vi "Set Run Control.vi"(8 "error in (no error)":errorcluster, 10 "Run Control":T1, 11 "PXIe5105 in":refnum<class "PXIe5105.lvclass">) -> (0 "error out":errorcluster, 3 "PXIe5105 out":refnum<class "PXIe5105.lvclass">)   [LabVIEW 2018, in "PXIe5105.lvlib" / "PXIe5105.lvclass"]
doc: "This Override method is used to set the Oscope instrument running mode. The 'Run Control' control has 3 modes of operation: 0-Run (or continuous), 1 - Single, 2 - Stop."
uses:
  PXIe5105.lvclass
  PPLs/Oscilloscope/Parent/Oscilloscope.lvlibp/Custom Controls/Run Control.ctl
  PXIe5105.lvclass/PXIe5105.ctl
  <instrlib>/niScope/Configure/Trigger/niScope Configure Trigger Software.vi
  PPLs/Oscilloscope/Parent/Oscilloscope.lvlibp
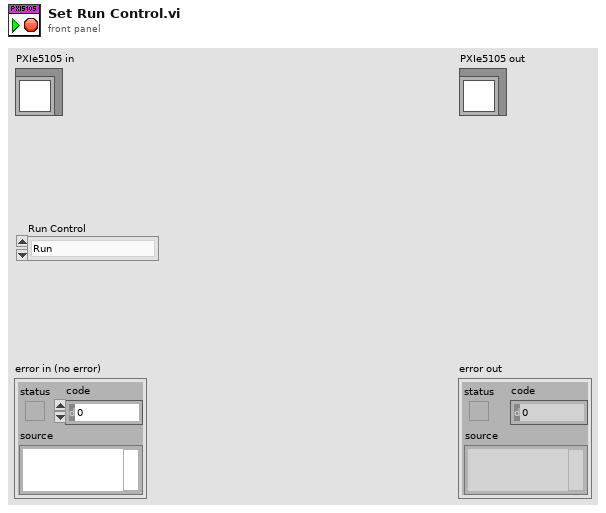
[diagram p1: front panel]
types:
  T1 = typedef "Oscilloscope.lvlibp/Run Control.ctl" = enum16{"Run", "Single", "Stop"}
  T2 = typedef "Oscilloscope.lvlibp/Analog Channels.ctl" = enum16{"1", "2", "3", "4", "5", "6", "7", "8", "9", "10", "11", "12", "13", "14", "15", "16"}
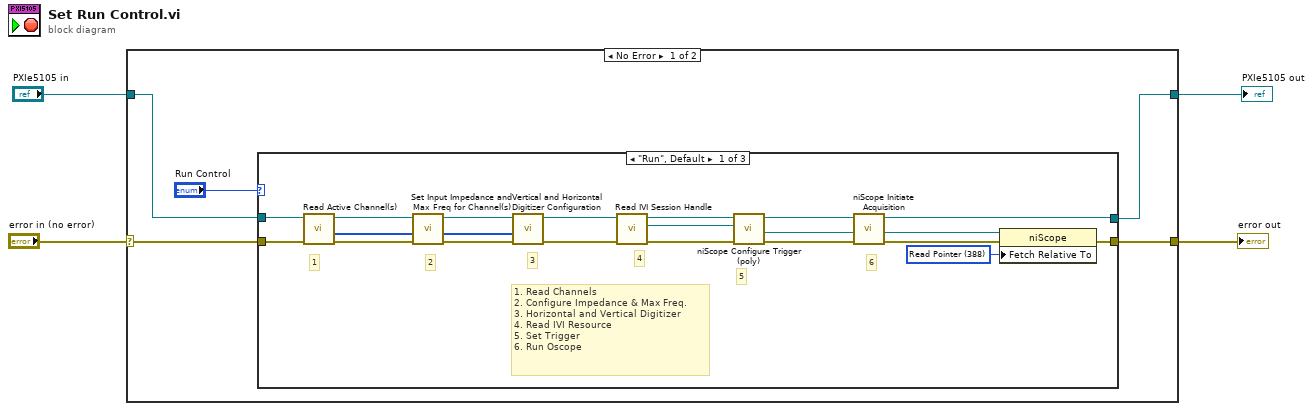
[diagram p0: block diagram]
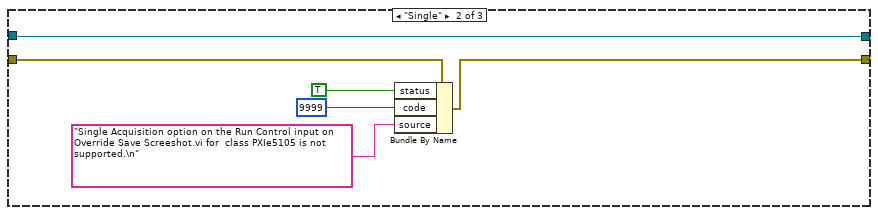
[diagram p2: hidden frame]
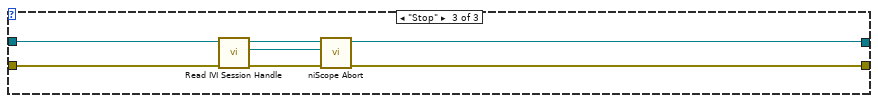
[diagram p3: hidden frame]
diagram:
  n1 = case shown="No Error" "error in (no error)" {
    selector: "error in (no error)" -> [w7 w41]
    tunnel: [w8 w41] -> w3
    tunnel: [w5 w40] -> w2
    tunnel: "PXIe5105 in" -> [w6 w40]
    frame No Error {
      n2 = case shown="\"Run\", Default" "Run Control" {
        tunnel: w7 -> [w26 w30 w36]
        tunnel: [w12 w29 w39] -> w8
        tunnel: w6 -> [w27 w28 w38]
        tunnel: [w19 w28 w34] -> w5
        frame "Run", Default {
          w15 = 388 items=["Start"=482, "Trigger"=483, "Pretrigger"=477, "Now"=481, "Read Pointer"=388] ("Fetch:Fetch Relative To")
          # "6"
          # "1. Read Channels\n2. Configure Impedance & Max Freq.\n3. Horizontal and Vertical Digitizer\n4. Read IVI Resource\n5. Set Trigger\n6. Run Oscope"
          # "5"
          # "4"
          # "3"
          # "2"
          # "1"
          n3 = call "Read Active Channel(s).vi"("error in (no error)"=w26, "PXIe5105 in"=w27) -> ("error out"=w25:errorcluster, "Active Channel(s)"=w18:T2[], "PXIe5105 out"=w23:refnum<class "PXIe5105.lvclass">)  [unwired: 7 in]
          n4 = call "Set Input Impedance and Max Freq for Channel(s).vi"("Channel(s)"=w18, "error in (no error)"=w25, "PXIe5105 in"=w23) -> ("error out"=w24:errorcluster, "PXIe5105 out"=w22:refnum<class "PXIe5105.lvclass">)  [unwired: 7 in]
          n5 = call "Vertical and Horizontal Digitizer Configuration.vi"("Channel(s)"=w18, "error in (no error)"=w24, "PXIe5105 in"=w22) -> ("error out"=w20:errorcluster, "PXIe5105 out"=w21:refnum<class "PXIe5105.lvclass">)  [unwired: 7 in]
          n6 = call "Read IVI Session Handle.vi"("error in (no error)"=w20, "PXIe5105 in"=w21) -> ("error out"=w16:errorcluster, "IVI Session Handle"=w17:refnum<k15>, "PXIe5105 out"=w19:refnum<class "PXIe5105.lvclass">)  [unwired: 7 in]
          n7 = call-poly <instrlib>:"niScope Configure Trigger (poly).vi"("instrument handle"=w17, "error in"=w16) -> ("instrument handle out"=w11:refnum<k15>, "error out"=w14:errorcluster)  [unwired: 12 in]
          n8 = call <instrlib>:"niScope Initiate Acquisition.vi"("instrument handle"=w11, "error in"=w14) -> ("instrument handle out"=w10:refnum<k15>, "error out"=w13:errorcluster)  [unwired: 12 in]
          n9 = property class="niScope"(reference=w10, error in=w13, "Fetch Relative To"=w15) -> (error out=w12:errorcluster)  [unwired: 1 out]
        }
        frame "Single" {
          n10 = Bundle By Name(cluster=w30, "status"=TRUE, "code"=9999, "source"="Single Acquisition option on the Run Control input on Override Save Screeshot.vi for  class PXIe5105 is not supported.\n") -> (w29:errorcluster)
        }
        frame "Stop" {
          n11 = call "Read IVI Session Handle.vi"("error in (no error)"=w36, "PXIe5105 in"=w38) -> ("error out"=w35:errorcluster, "IVI Session Handle"=w37:refnum<k15>, "PXIe5105 out"=w34:refnum<class "PXIe5105.lvclass">)  [unwired: 7 in]
          n12 = call <instrlib>:"niScope Abort.vi"("instrument handle"=w37, "error in"=w35) -> ("error out"=w39:errorcluster)  [unwired: 12 in, 1 out]
        }
      }
    }
    frame Error {
    }
  }
  "error out" <- w3
  "PXIe5105 out" <- w2
